vi "CalcArea.vi"(8 "Error In":errorcluster, 11 "Figure in":refnum<class "Figure.lvclass">) -> (0 "Error Out":errorcluster, 2 "Area":dbl, 3 "Figure out":refnum<class "Figure.lvclass">)   [LabVIEW 2021, in "Figure.lvclass"]
doc: "Calc a area - abstract class."
uses:
  Figure.lvclass
  <vilib>/Utility/error.llb/Error Cluster From Error Code.vi
  <vilib>/ErrorRing/Error Ring.xnode
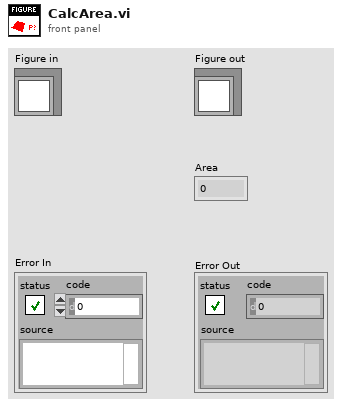
[diagram p1: front panel]
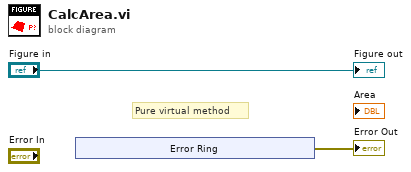
[diagram p0: block diagram]
diagram:
  # "Pure virtual method"
  n1 = xnode "Error Ring"() -> ("error out"=→"Error Out":errorcluster)
  "Figure out" <- "Figure in"
